vi "CO Serial CAL & Data Recording & DECADEv3.3_test.vi"() -> ()   [LabVIEW 2014]
uses:
  <vilib>/Platform/TimedLoop/XDataNode/timing_clust.ctl
  <vilib>/Platform/TimedLoop/XDataNode/nitl_modes.ctl
  <vilib>/Platform/TimedLoop/XDataNode/wakeup.ctl
  C:/Program Files (x86)/National Instruments/LabVIEW 2014/examples/Data Communication/Network Streams/Simple Network Streams/support/Network Stream Command.ctl
  <vilib>/Utility/error.llb/whitespace.ctl
  <vilib>/Instr/_visa.llb/VISA Configure Serial Port (Instr).vi
  <vilib>/Utility/tcp.llb/UDP Multicast Write-Only Open.vi
  <vilib>/platform/TimedLoop/XDataNode/XDataNode.xnode
  <vilib>/Platform/TimedLoop/XDataNode/XDNodeRunTimeDep.lvlib
panel:
  out "Stop File Write":bool
  out "Default file name":string
  in  "Flight Number 2":string="XXXX"
  out "status":bool
  out "CO Vacuum":bool
  out "CO CAL":bool
  out "error out":errorcluster
  out "CO Vacuum?":i16
  out "Control data":i32[](array[numeric])
  out "Control data out":string
  in  "VISA resource name":refnum<visa-resource-name>="ASRL8::INSTR"
  out "Serial VISA error":errorcluster
  out "SEPTIC TCP Error Out":errorcluster
  out "TCP packet\nSend To SEPTIC":bool
  in  "msec to wait":u32=330 caption="mSec to Wait"
  in  "UDP Time Stamp\nOffset":u32=1
  out "Scan from String Error \nCounter from process loop":i32
  out "TCP Binary Packet":string
  in  "ue9LJ temp":u16
  out "FISH TCP Error Out":errorcluster
  out "TCP packet\nSend To FISH":bool
  out "UDP_Out_Error Out":errorcluster
  out "Data Array":string[](array[string])
  out "UDP_Out Status":bool
  out "Data Process Status":bool
  out "Command In":string[](array[string])
  out "ERR Counter":i32
  out "UDP_Out":string
  out "UDP_Pack_num":u32
  out "Flight Number":string
  in  "aux":string="0"
  in  "acs2653pc_hdd":string="0"
  in  "LabviewVIclient vn":string="0"
  in  "LabviewVIserver vn":string="0"
  in  "PTP Sync":string="0"
  out "OK RAW COUNTER":i32
  out "IN_CAL?":bool
  out "Redundent DATA":string
  out "Data String":string
  out "CO_Data_Buffer":string[](array[string])
  out "RAW DATA":string
  out "loop count":i32
  out "Number of Read error":i32
  out "Command In":string
  # "Pre-flight"
  # "CONC"
  # "SIG"
  # "SENS"
  # "ZERO"
  # "Lamp flow controller"
  # "Lamp temperature"
  # "Monochromater flow controller"
  # "Monochromater temperature"
  # "Monochromater pressure"
  # "Fluorescence cell pressure"
  # "Calibration gas pressure"
  # "Cell temperature"
  # "Calibration Concentration"
  # "ERROR number"
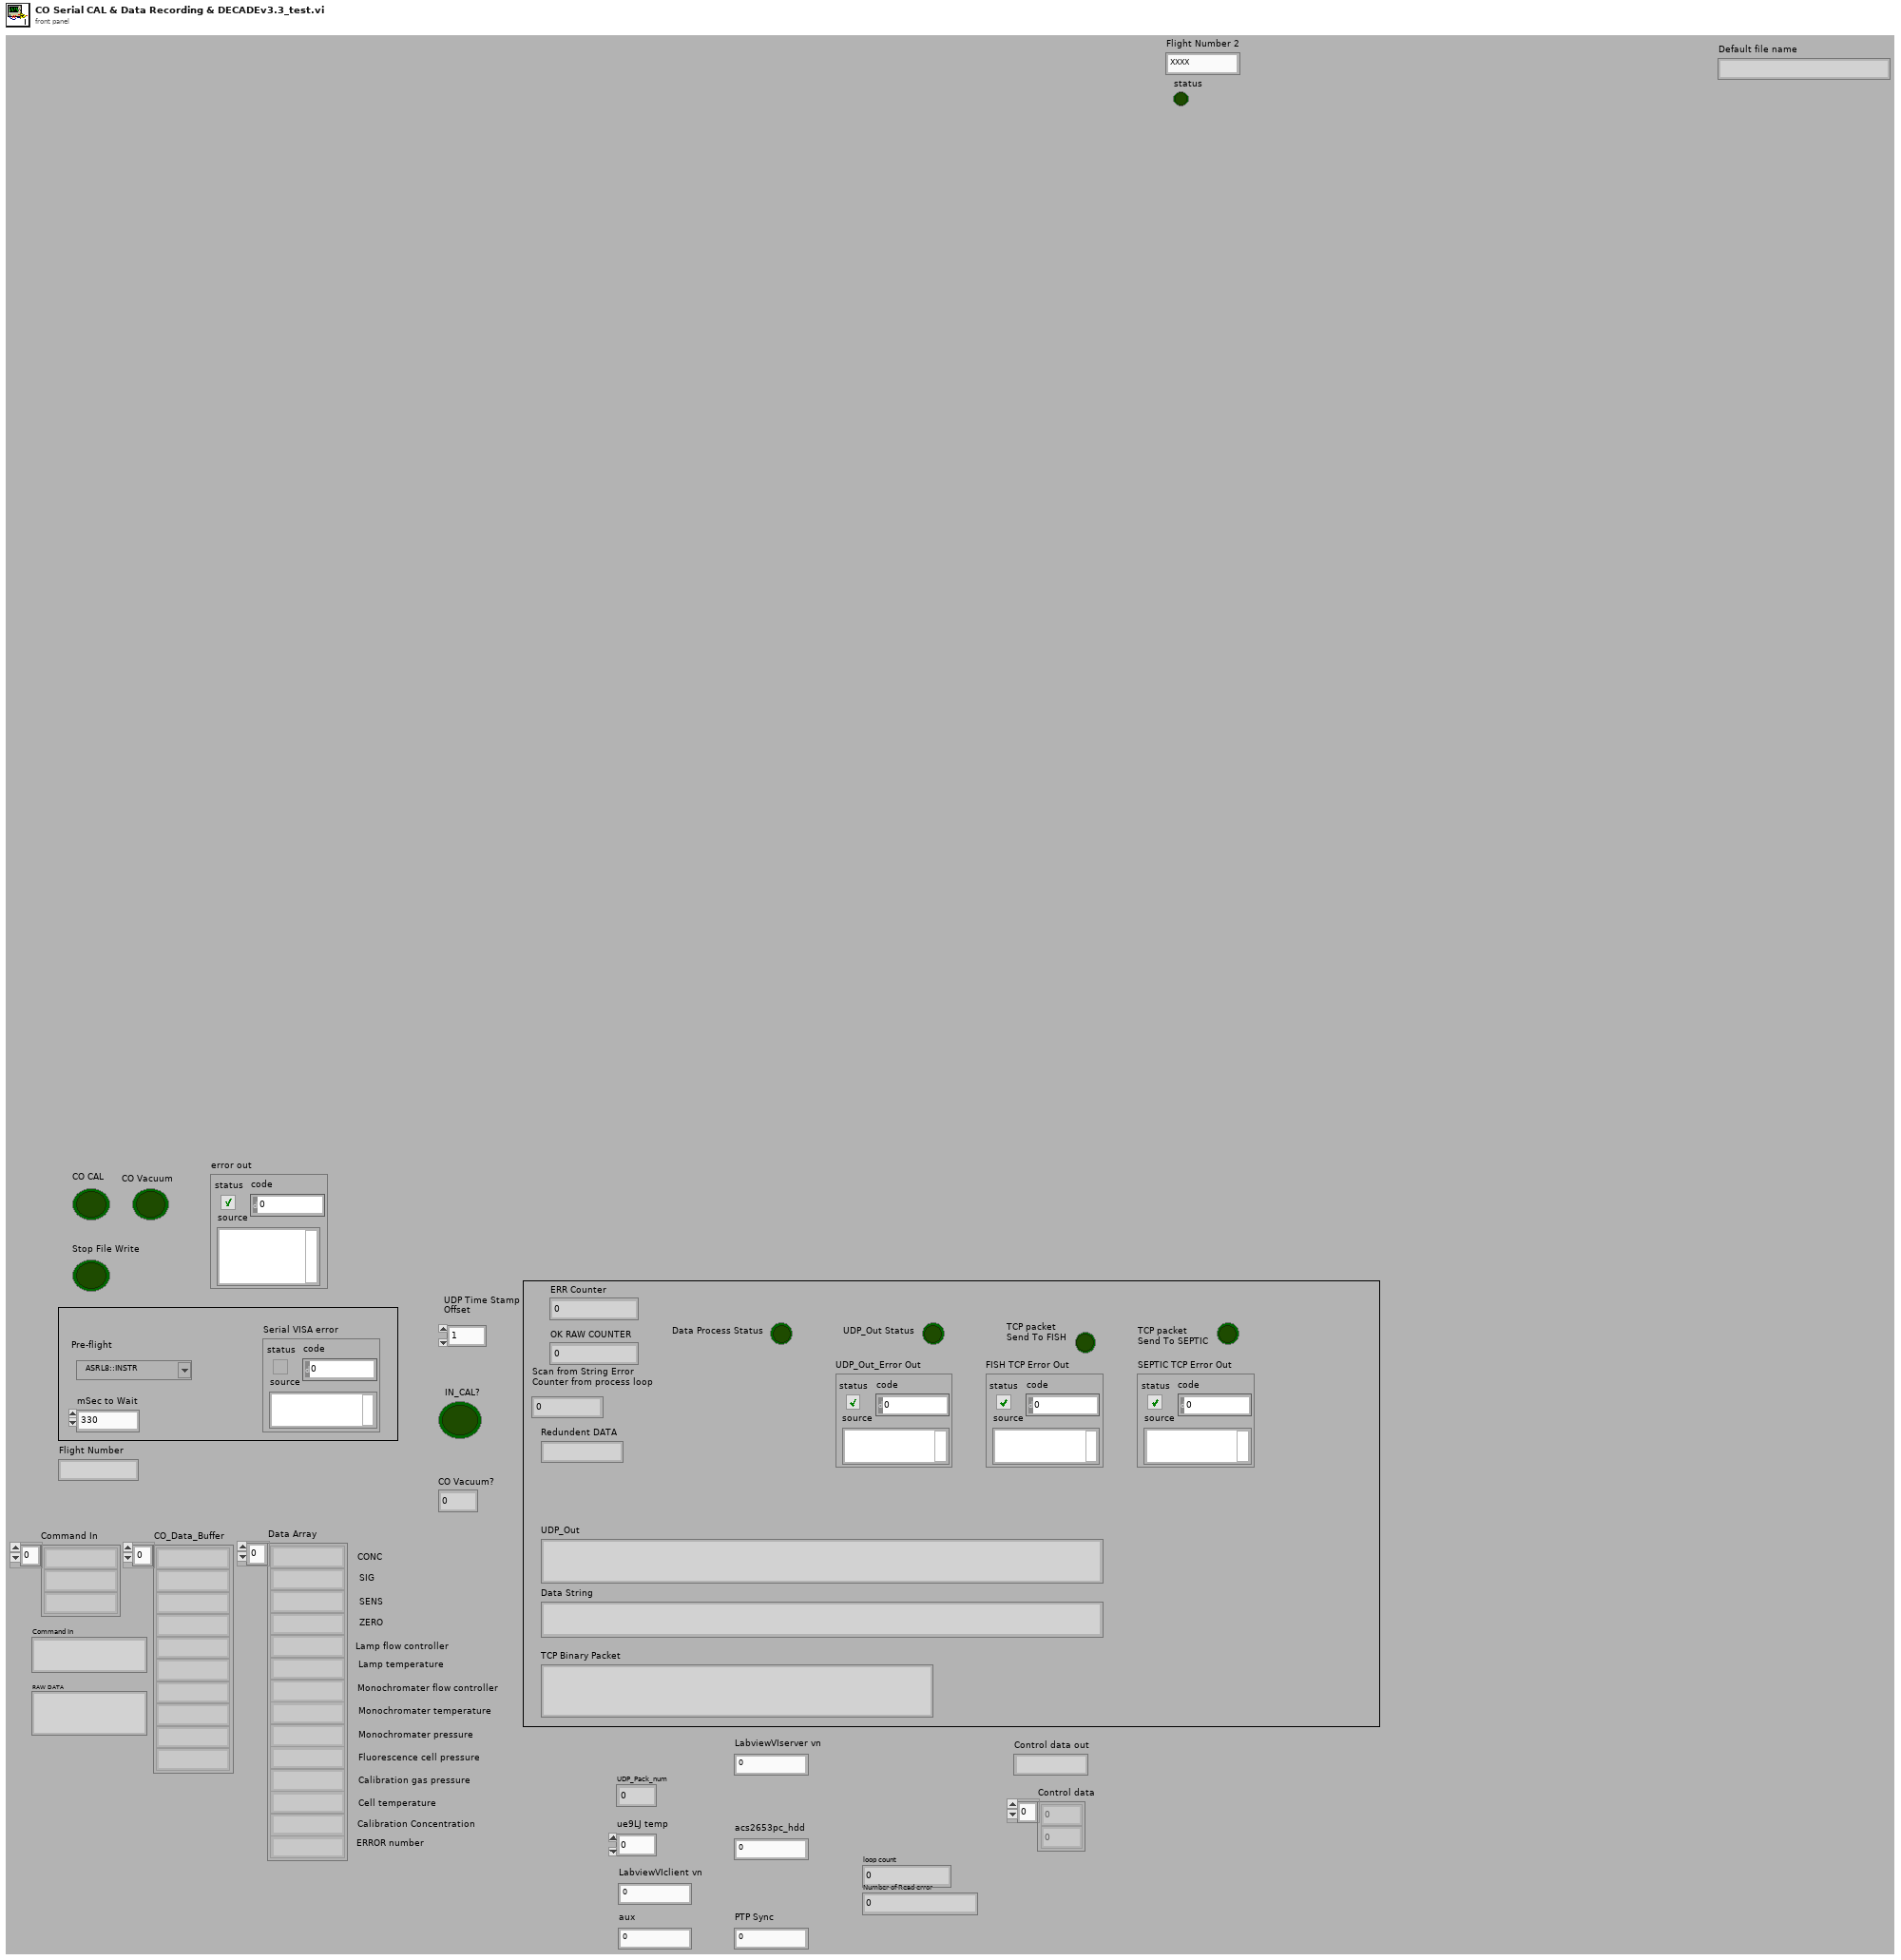
[diagram p1: front panel]
types:
  T1 = typedef "XDNodeRunTimeDep.lvlib/timing_clust.ctl" = cluster{"Expected End [f-1]":u64, "Actual End [f-1]":u64, "Finished Late? [f-1]":bool, "Expected End [i-1]":u64, "Actual End [i-1]":u64, "Finished Late? [i-1]":bool, "Expected Start [i]":u64, "Actual Start [i]":u64, "Expected Start [f]":u64, "Actual Start [f]":u64, "Source Name":string, "Structure Name":string, "Period":i64, "Deadline":i64, "Offset":i64, "Start":i64, "Priority":i32, "Timeout":i32, "Mode":T2, "Wakeup Reason":T3, "Error":errorcluster, "Source Type":string, "Secondary Source Type":string, "Global End Time":u64, "Global Start Time":u64, "Frame Duration":u64, "Iteration Duration":u64, "Assigned CPU":i32, "I/O Scan Engine Mode":u32}
  T2 = typedef "XDNodeRunTimeDep.lvlib/nitl_modes.ctl" = enum32{"No Change", "Process missed periods, maintain original phase", "Discard missed periods, maintain original phase", "Process missed periods, ignore original phase", "Discard missed periods, ignore original phase"}
  T3 = typedef "XDNodeRunTimeDep.lvlib/wakeup.ctl" = enum32{"Normal", "Aborted", "Asynchronous wakeup", "Timing source error", "Timed loop error", "Timeout"}
  T4 = typedef "Network Stream Command.ctl" = cluster{"Message":string, "Message Data":variant}
  T5 = enum16{"open", "replace", "create", "open or create", "replace or create", "replace or create with confirmation"}
  T6 = typedef "whitespace.ctl" = u16
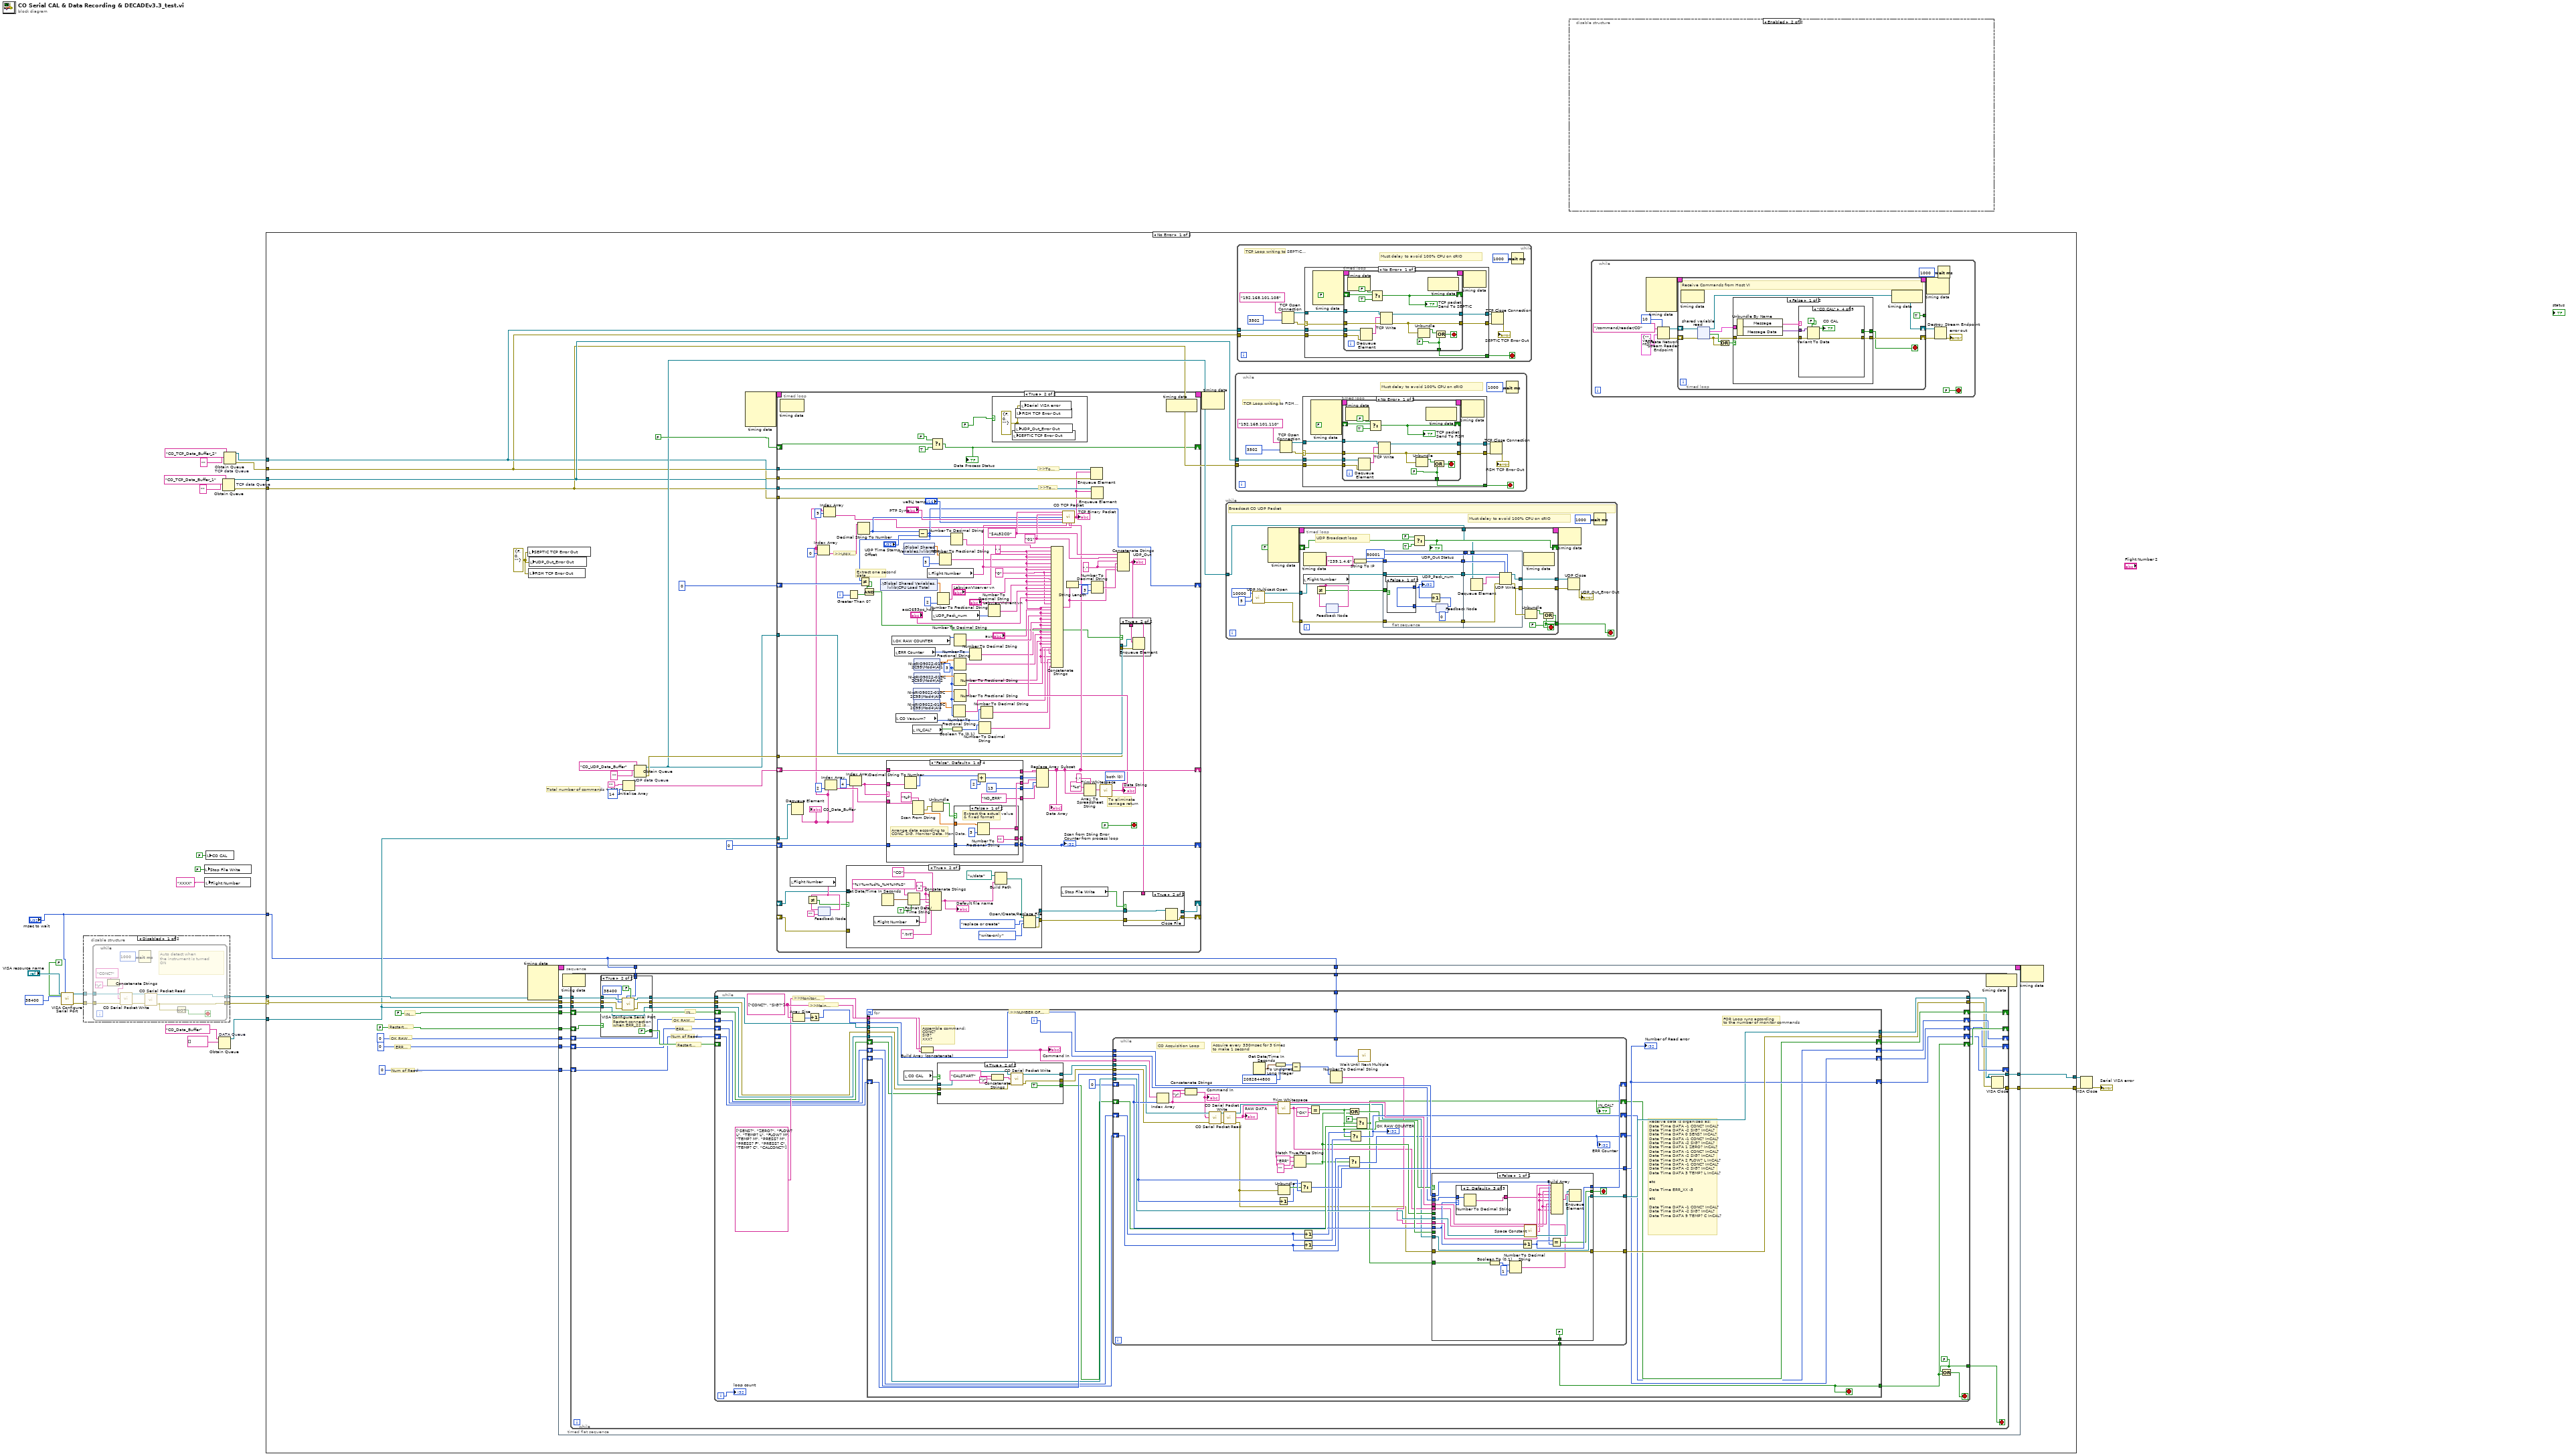
[diagram p0: block diagram]
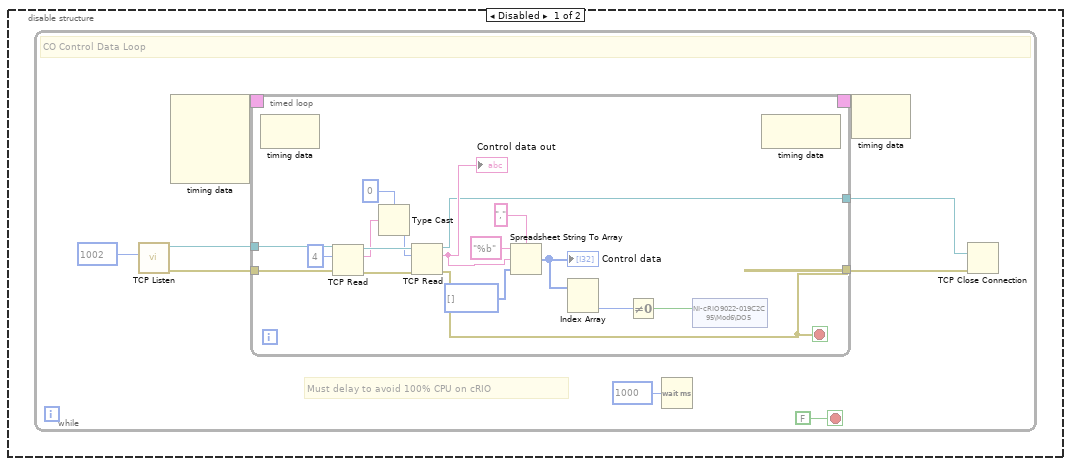
[diagram p3: hidden frame]
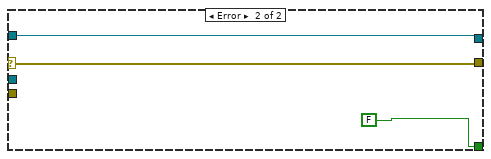
[diagram p4: hidden frame]
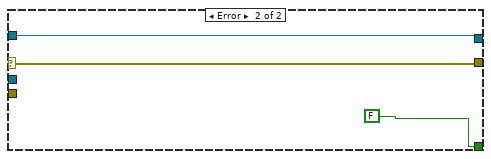
[diagram p5: hidden frame]
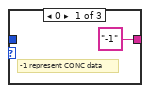
[diagram p7: hidden frame]
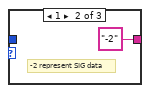
[diagram p8: hidden frame]
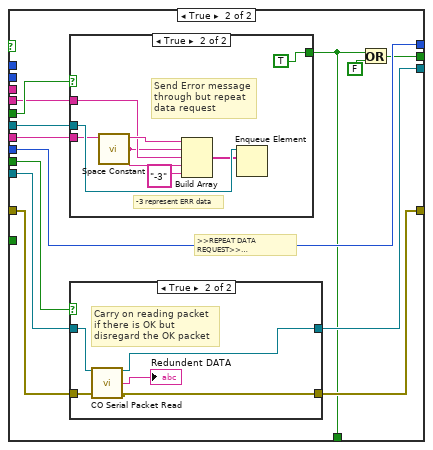
[diagram p9: hidden frame]
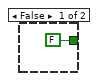
[diagram p11: hidden frame]
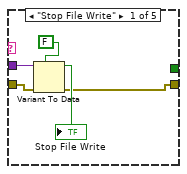
[diagram p13: hidden frame]
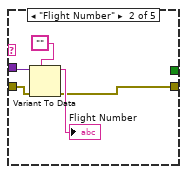
[diagram p14: hidden frame]
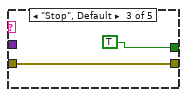
[diagram p15: hidden frame]
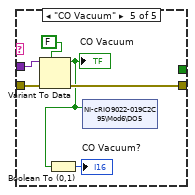
[diagram p16: hidden frame]
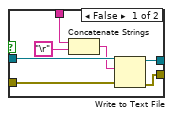
[diagram p19: hidden frame]
diagram:
  n1 = call-poly "VISA Configure Serial Port"("VISA resource name"="VISA resource name", "timeout (10sec)"="msec to wait", "Enable Termination\nChar (T)"=FALSE ("Enable Termination\nChar (T)"), "baud rate (9600)"=u32 38400) -> ("VISA resource name out"=w12:refnum<visa-resource-name>, "error out"=w11:errorcluster)  [unwired: 10 in]
  n2 = disable-structure shown="Disabled" {
    disable-tunnel: w12 -> [w29 _]
    disable-tunnel: w11 -> [w28 _]
    disable-tunnel: [w27 _] -> w10
    disable-tunnel: [w26 _] -> w9
    frame Disabled {
      n3 = while {
        tunnel: w29 -> [w40]
        tunnel: w28 -> [w39]
        tunnel: [w33] -> w27
        tunnel: [w34] -> w26
        stop <- w38 stop-if-true
        # "Auto detect when\nthe instrument is turned \nON"
        n4 = Concatenate Strings("CONC?" ("Data in"), "\r") -> (w30:string)
        n5 = call "CO Serial Packet Write.vi"("VISA resource name In"=w40, "Data in"=w30, "error in (no error)"=w39) -> ("VISA resource name Out"=w36:refnum<visa-resource-name>, "error out"=w35:errorcluster)  [unwired: 11 in]
        n6 = Wait (ms)(milliseconds to wait=u32 1000) -> ()  [unwired: 1 out]
        n7 = call "CO Serial Packet Read.vi"("VISA resource In"=w36, "error in"=w35) -> ("VISA resource Out"=w33:refnum<visa-resource-name>, "error out"=w34:errorcluster)  [unwired: 11 in, 1 out]
        n8 = Not(x=w34) -> (.not. x?=w38:bool)
      }
    }
    frame Enabled {
    }
  }
  n9 = local write "Stop File Write"(FALSE ("Stop File Write")) -> ()
  n10 = local write "Flight Number"("XXXX" ("Flight Number")) -> ()
  n11 = local write "CO CAL"(FALSE ("CO CAL")) -> ()
  n12 = Obtain Queue "DATA Queue"(name (unnamed)="CO_Data_Buffer", element data type=string[] []) -> (queue out=w23:refnum<queue>)  [unwired: 3 in, 2 out]
  n13 = Obtain Queue "TCP data Queue"(name (unnamed)="CO_TCP_Data_Buffer_1", element data type="") -> (queue out=w22:refnum<queue>, error out=w21:errorcluster)  [unwired: 3 in, 1 out]
  n14 = Obtain Queue "TCP data Queue"(name (unnamed)="CO_TCP_Data_Buffer_2", element data type="") -> (queue out=w20:refnum<queue>, error out=w19:errorcluster)  [unwired: 3 in, 1 out]
  n15 = case shown="No Error" w9 {
    selector: w9 -> [w68 w697]
    tunnel: w10 -> [w69 w696]
    tunnel: [w70 w697] -> w15
    tunnel: [w46 w696] -> w14
    tunnel: w23 -> [w67 _]
    tunnel: w22 -> [w56 _]
    tunnel: w21 -> [w55 _]
    tunnel: w20 -> [w54 _]
    tunnel: w19 -> [w53 _]
    tunnel: "msec to wait" -> [w41 _]
    frame No Error {
      w52 = errorcluster {"status"=FALSE, "code"=0, "source"=""} ("UDP_Out_Error Out")
      # "Restart connection?"
      # "IN CAL?"
      # "OK RAW Counter"
      # "ERR Counter"
      # "Num of Read Error"
      # "Total number of commands + ERR"
      n16 = node-c288() -> (w43:T1)  [unwired: 4 in]
      n17 = local write "SEPTIC TCP Error Out"(w52) -> ()
      n18 = local write "FISH TCP Error Out"(w52) -> ()
      n19 = local write "UDP_Out_Error Out"(w52) -> ()
      n20 = timed-sequence {
        timing: w43 -> [_]
        timing-out: [_] -> w42
        tunnel: [w166] -> w70
        tunnel: w69 -> [w165]
        tunnel: w68 -> [w164]
        tunnel: w67 -> [w163]
        tunnel: FALSE -> [w162]
        tunnel: 0 -> [w161]
        tunnel: 0 -> [w160]
        tunnel: 0 -> [w159]
        tunnel: FALSE ("IN_CAL?") -> [w158]
        tunnel: [w157] -> w46
        tunnel: w41 -> [w156]
        tunnel: w41 -> [w155]
        n21 = timed-flat-sequence {
          tunnel: [w178] -> w166
          tunnel: w165 -> [w177]
          tunnel: w164 -> [w176]
          tunnel: w163 -> [w175]
          tunnel: w162 -> [w174]
          tunnel: w161 -> [w173]
          tunnel: w160 -> [w172]
          tunnel: w159 -> [w171]
          tunnel: w158 -> [w170]
          tunnel: [w169] -> w157
          tunnel: w156 -> [w168]
          tunnel: w155 -> [w167]
          n22 = node-c288() -> ()  [unwired: 1 in, 1 out]
          n23 = while {
            tunnel: [w183] -> w178
            tunnel: w177 -> [w200]
            tunnel: w176 -> [w199]
            tunnel: w175 -> [w197]
            shift-right: [w194] -> _
            shift-left: w174 -> [w195]
            shift-right: [w190] -> _
            shift-left: w173 -> [w191]
            shift-right: [w187] -> _
            shift-left: w172 -> [w189]
            shift-right: [w186] -> _
            shift-left: w171 -> [w188]
            shift-right: [w184] -> _
            shift-left: w170 -> [w185]
            tunnel: [w181] -> w169
            tunnel: w168 -> [w180]
            tunnel: w167 -> [w179]
            stop <- w193 stop-if-true
            # "Restart connection?"
            # "Num of Read Error"
            # "ERR Counter"
            # "IN CAL?"
            # "OK RAW Counter"
            n24 = case shown="True" w195 {
              selector: w195 -> [w202 _]
              tunnel: [w205 w211] -> w201
              tunnel: w200 -> [w205 w212]
              tunnel: [w204 w210] -> w198
              tunnel: w199 -> [w204 w209]
              tunnel: [w203 w214] -> w196
              tunnel: w197 -> [w203 w214]
              tunnel: [w202 FALSE] -> w192
              tunnel: w179 -> [_ w206]
              frame False {
              }
              frame True {
                # "Restart connection\nwhen ERR_22 is detected"
                n25 = call-poly "VISA Configure Serial Port"("VISA resource name"=w212, "timeout (10sec)"=w206, "Enable Termination\nChar (T)"=FALSE ("Enable Termination\nChar (T)"), "baud rate (9600)"=u32 38400, "error in (no error)"=w209) -> ("VISA resource name out"=w211:refnum<visa-resource-name>, "error out"=w210:errorcluster)  [unwired: 9 in]
              }
            }
            n26 = while {
              tunnel: [w236] -> w182
              tunnel: w201 -> [w235]
              tunnel: w198 -> [w234]
              tunnel: [w233] -> w181
              tunnel: w196 -> [w232]
              shift-right: [w223] -> w190
              shift-left: w191 -> [w227]
              shift-right: [w222] -> w187
              shift-left: w189 -> [w226]
              shift-right: [w221] -> w184
              shift-left: w185 -> [w225]
              shift-right: [w220] -> w186
              shift-left: w188 -> [w224]
              tunnel: [w216] -> w193
              shift-right: [w217] -> w194
              shift-left: w192 -> [_]
              tunnel: w180 -> [w215]
              i -> [w219]
              stop <- w218 stop-if-true
              w216 = FALSE
              w231 = string[] ["CONC?", "SIG?"]
              # ">>Main commands>>"
              # ">>Monitor Command>>"
              n27 = Array Size(array=w231) -> (size(s)=w228:i32)
              n28 = Increment(x=w228) -> (x+1=w230:i32)
              n29 = for {
                tunnel: w235 -> [w256]
                tunnel: w234 -> [w255]
                tunnel: [w261] -> w236
                shift-right: [w259] -> w220
                shift-left: w224 -> [w260]
                tunnel: [w258] -> w233
                tunnel: w232 -> [w257]
                tunnel: w230 -> [w251]
                shift-right: [w249] -> w221
                shift-left: w225 -> [w250]
                shift-right: [w247] -> w222
                shift-left: w226 -> [w248]
                shift-right: [w245] -> w223
                shift-left: w227 -> [w246]
                tunnel: string[] ["SENS?", "ZERO?", "FLOW? L", "TEMP? L", "FLOW? M", "TEMP? M", "PRESS? M", "PRESS? F", "PRESS? C", "TEMP? C", "CALCONC?"] -> [w242] mode=indexing
                tunnel: w231 -> [w243]
                tunnel: [w240] -> w217
                tunnel: w215 -> [w238]
                i -> [w241]
                stop <- w240 stop-if-true
                # "Receive data is organised as:\nDate Time DATA -1 CONC? InCAL?\nDate Time DATA -2 SIG? InCAL?\nDate Time DATA 0 SENS? InCAL?\nDate Time DATA -1 CONC? InCAL?\nDate Time DATA -2 SIG? InCAL?\nDate Time DATA 1 ZERO? InCAL?\nDate Time DATA -1 CONC? InCAL?\nDate Time DATA -2 SIG? InCAL?\nDate Time DATA 2 FLOW? L InCAL?\nDate Time DATA -1 CONC? InCAL?\nDate Time DATA -2 SIG? InCAL?\nDate Time DATA 3 TEMP? L InCAL?\n\netc\n\nDate Time ERR_XX -3\n\netc\n\nDate Time DATA -1 CONC? InCAL?\nDate Time DATA -2 SIG? InCAL?\nDate Time DATA 9 TEMP? C InCAL?"
                # "FOR Loop runs according\nto the number of monitor commands"
                # "Assemble command:\nCONC?\nSIG?\nXXX?"
                # ">>NUMBER OF COMMANDS>>"
                n30 = local read "CO CAL"() -> (w237:bool)
                n31 = Build Array (concatenate)(w243, w242) -> (w244:string[])
                "Command In" <- w244
                n32 = case shown="True" w237 {
                  tunnel: w256 -> [w361 w363]
                  tunnel: w255 -> [w360 w366]
                  tunnel: [w361 w364] -> w254
                  tunnel: [w360 w365] -> w253
                  tunnel: [w359 TRUE ("IN_CAL?")] -> w252
                  tunnel: w250 -> [w359 _]
                  frame False {
                  }
                  frame True {
                    n33 = Concatenate Strings("CALSTART" ("string"), "\r") -> (w362:string)
                    n34 = call "CO Serial Packet Write.vi"("VISA resource name In"=w363, "Data in"=w362, "error in (no error)"=w366) -> ("VISA resource name Out"=w364:refnum<visa-resource-name>, "error out"=w365:errorcluster)  [unwired: 11 in]
                  }
                }
                n35 = while {
                  tunnel: w253 -> [w268]
                  tunnel: [w295] -> w261
                  tunnel: w260 -> [w307]
                  tunnel: [w306] -> w259
                  tunnel: w244 -> [w299]
                  tunnel: [w296] -> w258
                  tunnel: w257 -> [w294]
                  tunnel: w254 -> [w270]
                  shift-right: [w271] -> w249
                  shift-left: w252 -> [w301]
                  shift-right: [w298] -> _
                  shift-left: 0 -> [w300]
                  tunnel: w251 -> [w291]
                  shift-right: [w288] -> w247
                  shift-left: w248 -> [w289]
                  shift-right: [w282] -> w245
                  shift-left: w246 -> [w284]
                  tunnel: w241 -> [w281]
                  tunnel: [w276] -> w240
                  tunnel: w238 -> [w262]
                  stop <- w297 stop-if-true
                  # "Acquire every 330msec for 3 times\nto make 1 second"
                  # "CO Acquisition Loop"
                  n36 = Index Array(array=w299, index=w300) -> (element=w293:string)
                  n37 = Concatenate Strings(w293, "\r") -> (w269:string)
                  "Command In" <- w269
                  n38 = call "CO Serial Packet Write.vi"("VISA resource name In"=w270, "Data in"=w269, "error in (no error)"=w268) -> ("VISA resource name Out"=w266:refnum<visa-resource-name>, "error out"=w267:errorcluster)  [unwired: 11 in]
                  n39 = call "CO Serial Packet Read.vi"("VISA resource In"=w266, "error in"=w267) -> ("VISA resource Out"=w265:refnum<visa-resource-name>, "Data Out"=w263:string, "error out"=w264:errorcluster)  [unwired: 11 in]
                  "RAW DATA" <- w263
                  n40 = Get Date/Time In Seconds() -> (seconds since 1Jan1904=w277:timestamp)
                  n41 = To Unsigned Long Integer(number=w277) -> (unsigned 32bit integer=w280:u32)
                  n42 = Increment(x=w307) -> (x+1=w303:i32)
                  n43 = call <vilib>:"Trim Whitespace.vi"("string"=w263) -> ("trimmed string"=w275:string)  [unwired: 1 in]
                  n44 = Unbundle(w264) -> ("status"=w304:bool)  [unwired: 2 out]
                  n45 = Subtract(x=w280, y=u32 2082844800) -> (x-y=w272:u32)
                  n46 = Match True/False String(2:"" ("false string"), 3:"ERR" ("true string"), 4:w263) -> (0:w283:bool)  [unwired: 1 out]
                  n47 = Select(t=w303, s=w304, f=w307) -> (s? t:f=w306:i32)
                  n48 = Increment(x=w289) -> (x+1=w290:i32)
                  n49 = Increment(x=w284) -> (x+1=w285:i32)
                  n50 = Equal?(x=w275, y="OK" ("string")) -> (x = y?=w286:bool)
                  n51 = Number To Decimal String(number=w272) -> (decimal integer string=w278:string)  [unwired: 1 in]
                  n52 = Select(t=w285, s=w283, f=w284) -> (s? t:f=w282:i32)
                  "ERR Counter" <- w282
                  n53 = Select(t=w290, s=w286, f=w289) -> (s? t:f=w288:i32)
                  "OK RAW COUNTER" <- w288
                  n54 = Compound Arithmetic op=OR(w286, w283) -> (w287:bool)
                  n55 = Select(t=FALSE, s=w286, f=w301) -> (s? t:f=w271:bool)
                  "IN_CAL?" <- w271
                  n56 = call "Wait Until Next Multiple"("Count(mSec)"=w262) -> ()  [unwired: 1 out]
                  n57 = case shown="False" w287 {
                    tunnel: w300 -> [w315 w343]
                    tunnel: [w326 w343] -> w298
                    tunnel: [w320 w333] -> w297
                    tunnel: w265 -> [w325 w342]
                    tunnel: w264 -> [w324 w341]
                    tunnel: [w325 w340] -> w296
                    tunnel: [w324 w339] -> w295
                    tunnel: w294 -> [w322 w337]
                    tunnel: w275 -> [w313 w335]
                    tunnel: w293 -> [w316 _]
                    tunnel: w278 -> [w321 w336]
                    tunnel: w283 -> [_ w338]
                    tunnel: w291 -> [w319 _]
                    tunnel: w286 -> [_ w334]
                    tunnel: w281 -> [w318 _]
                    tunnel: [FALSE w331] -> w276
                    tunnel: w271 -> [w312 _]
                    frame False {
                      n58 = case shown="2, Default" w315 {
                        tunnel: w318 -> [_ _ w330]
                        tunnel: ["-1" "-2" w329] -> w317
                        frame 0 {
                          # "-1 represent CONC data"
                        }
                        frame 1 {
                          # "-2 represent SIG data"
                        }
                        frame 2, Default {
                          n59 = Number To Decimal String(number=w330) -> (decimal integer string=w329:string)  [unwired: 1 in]
                        }
                      }
                      n60 = Boolean To (0,1)(Boolean=w312) -> (0, 1=w311:i16)
                      n61 = Number To Decimal String(number=w311, width (-)=i16 1) -> (decimal integer string=w308:string)
                      n62 = Increment(x=w315) -> (x+1=w326:i32)
                      n63 = call <vilib>:"Space Constant.vi"() -> ("String"=w309:string)
                      n64 = Equal?(x=w326, y=w319) -> (x = y?=w320:bool)
                      n65 = Build Array(w321, w309, w313, w309, w317, w309, w316, w313, w309, w308) -> (w323:string[])
                      n66 = Enqueue Element(queue=w322, element=w323) -> ()  [unwired: 2 in, 3 out]
                    }
                    frame True {
                      # ">>REPEAT DATA REQUEST>>\nif OK or ERR"
                      n67 = case shown="True" w338 {
                        tunnel: w337 -> [_ w358]
                        tunnel: w336 -> [_ w356]
                        tunnel: w335 -> [_ w355]
                        tunnel: [FALSE TRUE] -> w331
                        frame False {
                        }
                        frame True {
                          # "-3 represent ERR data"
                          # "Send Error message\nthrough but repeat\ndata request"
                          n68 = call <vilib>:"Space Constant.vi"() -> ("String"=w354:string)
                          n69 = Build Array(w356, w354, w355, w354, "-3" ("element")) -> (w357:string[])
                          n70 = Enqueue Element(queue=w358, element=w357) -> ()  [unwired: 2 in, 3 out]
                        }
                      }
                      n71 = case shown="True" w334 {
                        tunnel: w342 -> [w344 w349]
                        tunnel: w341 -> [w345 w350]
                        tunnel: [w344 w348] -> w340
                        tunnel: [w345 w346] -> w339
                        frame False {
                        }
                        frame True {
                          # "Carry on reading packet\nif there is OK but\ndisregard the OK packet"
                          n72 = call "CO Serial Packet Read.vi"("VISA resource In"=w349, "error in"=w350) -> ("VISA resource Out"=w348:refnum<visa-resource-name>, "Data Out"=→"Redundent DATA":string, "error out"=w346:errorcluster)  [unwired: 11 in]
                        }
                      }
                      n73 = Or(x=w331, y=FALSE) -> (x .or. y?=w333:bool)
                    }
                  }
                }
                "Number of Read error" <- w259
              }
              n74 = Or(x=w216, y=w217) -> (x .or. y?=w218:bool)
              "loop count" <- w219
            }
            n75 = VISA Close(VISA resource name=w181, error in (no error)=w182) -> (error out=w183:errorcluster)
          }
          n76 = node-c288() -> ()  [unwired: 1 in, 1 out]
        }
      }
      n77 = Initialize Array("", 14) -> (w64:string[])
      n78 = Obtain Queue "UDP data Queue"(name (unnamed)="CO_UDP_Data_Buffer", element data type="") -> (queue out=w59:refnum<queue>, error out=w60:errorcluster)  [unwired: 3 in, 1 out]
      n79 = node-c288() -> (w45:T1)  [unwired: 4 in]
      n80 = timed-loop {
        tunnel: w67 -> [w530]
        shift-right: [w495] -> _
        shift-left: w64 -> [w513]
        shift-right: [w500] -> _
        shift-left: FALSE -> [w503]
        tunnel: w56 -> [w494]
        tunnel: w55 -> [w493]
        tunnel: w59 -> [w491]
        tunnel: w60 -> [w490]
        shift-right: [w488] -> _
        shift-left: 0 -> [w489]
        shift-right: [w474] -> _
        shift-left: 0 -> [w482]
        tunnel: w54 -> [w480]
        tunnel: w53 -> [w479]
        timing: w45 -> [_]
        timing-out: [_] -> w44
        shift-right: [w450] -> _
        shift-left: _ -> [w443]
        shift-right: [w441] -> _
        shift-left: _ -> [w442]
        i -> [w485]
        stop <- FALSE stop-if-true
        w431 = "0" ("string")
        w465 = i16 3 ("precision (6)")
        w505 = T6 0 items=["both", "start of string", "end of string"] ("location (both)")
        w438 = ","
        w498 = "01"
        w516 = ","
        w499 = "$AL52CO"
        # ">>To SEPTIC>>"
        # ">>To FISH>>"
        # "Extract one second data\nfor UDP sending"
        # ">>UNIX TIME>>"
        # "To eliminate\ncarriage return"
        n81 = node-c288() -> ()  [unwired: 1 in, 1 out]
        n82 = local read "Flight Number"() -> (w448:string)
        n83 = Dequeue Element(queue=w530) -> (element=w470:string[])  [unwired: 2 in, 3 out]
        "CO_Data_Buffer" <- w470
        n84 = Index Array(array=w470, index=0) -> (element=w483:string)
        n85 = feedback #1("" ("Flight Number")) -> (w447:string)
        n86 = Not Equal?(x=w448, y=w447) -> (x != y?=w446:bool)
        n87 = feedback-in #1(w448) -> ()
        n88 = Index Array(array=w470, index=9) -> (element=w469:string)
        n89 = Index Array(array=w470, index=2) -> (element=w511:string)
        n90 = case shown="True" w446 {
          tunnel: [w532 w534] -> w445
          tunnel: [w531 w533] -> w444
          tunnel: w443 -> [w532 _]
          tunnel: w442 -> [w531 _]
          frame False {
          }
          frame True {
            w541 = "_" ("string")
            n91 = local read "Flight Number"() -> (w547:string)
            n92 = Get Date/Time In Seconds() -> (seconds since 1Jan1904=w542:timestamp)
            n93 = Format Date/Time String(time format string (%c)="%Y%m%d%_%H%M%S", seconds (now)=w542, UTC format=TRUE) -> (date/time string=w545:string)
            n94 = Concatenate Strings("CO" ("string"), w541, w545, w541, w547, ".txt" ("string")) -> (w539:string)
            "Default file name" <- w539
            n95 = Build Path(base path=path "u:/data", name or relative path=w539) -> (appended path=w535:path)
            n96 = Open/Create/Replace File(file path (use dialog)=w535, operation (0:open)=T5."replace or create", access (0:read/write)=enum16{"read/write", "read-only", "write-only"}."write-only") -> (refnum out=w534:refnum<file>, error out=w533:errorcluster)  [unwired: 3 in, 1 out]
          }
        }
        n97 = Greater Than 0?(x=w485) -> (x > 0?=w484:bool)
        n98 = Index Array(array=w470, index=4) -> (element=w512:string)
        n99 = Decimal String To Number(string=w483) -> (number=w477:i32)  [unwired: 2 in, 1 out]
        n100 = shared-variable ".\\Global Shared Variables.lvlib\\CPU Load Total"() -> (w437:dbl)  [unwired: 1 in, 1 out]
        n101 = case shown="\"False\", Default" w512 {
          tunnel: w512 -> [w578 _ _ _]
          tunnel: w513 -> [w579 w601 w623 w637]
          tunnel: w511 -> [w570 w595 w617 w633]
          tunnel: [w579 w601 w623 w637] -> w510
          tunnel: [w576 0 ("index") 1 ("index") w634] -> w509
          tunnel: [w569 w591 w613 w633] -> w508
          tunnel: [w568 w592 w614 ""] -> _
          tunnel: w489 -> [w567 w594 w616 w635]
          tunnel: [w566 w593 w615 w635] -> w488
          tunnel: [13 ("index") 13 ("index") 13 ("index") w634] -> w473
          tunnel: ["NO_ERR" "NO_ERR" "NO_ERR" w633] -> w472
          frame "False", Default {
            # "Arrange data according to\nCONC, SIG, Monitor Data, Mon Data,"
            n102 = Decimal String To Number(string=w578) -> (number=w575:i32)  [unwired: 2 in, 1 out]
            n103 = Scan From String(format string="%f", input string=w570) -> (error out=w572:errorcluster, output 1=w573:dbl)  [unwired: 3 in, 2 out]
            n104 = Unbundle(w572) -> ("status"=w571:bool)  [unwired: 2 out]
            n105 = case shown="False" w571 {
              tunnel: [w584 ""] -> w569
              tunnel: w573 -> [w583 _]
              tunnel: w567 -> [w582 w587]
              tunnel: [w582 w586] -> w566
              tunnel: ["" "Scan from string error"] -> w568
              frame False {
                # "Extract the actual value\n& fixed format"
                n106 = Number To Fractional String(number=w583, precision (6)=i16 3) -> (F-format string=w584:string)  [unwired: 2 in]
              }
              frame True {
                # "If scan from string error,\nreplace data with empty\nstring"
                n107 = Increment(x=w587) -> (x+1=w586:i32)
              }
            }
            n108 = Add(x=w575, y=2) -> (x+y=w576:i32)
          }
          frame "-1" {
            # "Arrange data according to\nCONC, SIG, Monitor Data, Mon Data,"
            # "-1 represent CONC data"
            n109 = Scan From String(format string="%f", input string=w595) -> (error out=w597:errorcluster, output 1=w598:dbl)  [unwired: 3 in, 2 out]
            n110 = Unbundle(w597) -> ("status"=w596:bool)  [unwired: 2 out]
            n111 = case shown="False" w596 {
              tunnel: [w606 ""] -> w591
              tunnel: w598 -> [w605 _]
              tunnel: w594 -> [w604 w609]
              tunnel: [w604 w608] -> w593
              tunnel: ["" "Scan from string error"] -> w592
              frame False {
                # "Extract the actual value\n& fixed format"
                n112 = Number To Fractional String(number=w605, precision (6)=i16 5) -> (F-format string=w606:string)  [unwired: 2 in]
              }
              frame True {
                # "If scan from string error,\nreplace data with empty\nstring"
                n113 = Increment(x=w609) -> (x+1=w608:i32)
              }
            }
          }
          frame "-2" {
            # "Arrange data according to\nCONC, SIG, Monitor Data, Mon Data,"
            # "-2 represent SIG data"
            n114 = Scan From String(format string="%f", input string=w617) -> (error out=w619:errorcluster, output 1=w620:dbl)  [unwired: 3 in, 2 out]
            n115 = Unbundle(w619) -> ("status"=w618:bool)  [unwired: 2 out]
            n116 = case shown="False" w618 {
              tunnel: [w628 ""] -> w613
              tunnel: w620 -> [w627 _]
              tunnel: w616 -> [w626 w631]
              tunnel: [w626 w630] -> w615
              tunnel: ["" "Scan from string error"] -> w614
              frame False {
                # "Extract the actual value\n& fixed format"
                n117 = Number To Fractional String(number=w627, precision (6)=i16 3) -> (F-format string=w628:string)  [unwired: 2 in]
              }
              frame True {
                # "If scan from string error,\nreplace data with empty\nstring"
                n118 = Increment(x=w631) -> (x+1=w630:i32)
              }
            }
          }
          frame "-3" {
            w634 = 13 ("index")
            # "-3 represent ERR data"
          }
        }
        "Scan from String Error \nCounter from process loop" <- w488
        n119 = local read "OK RAW COUNTER"() -> (w514:i32)
        n120 = local read "ERR Counter"() -> (w453:i32)
        n121 = local read "CO Vacuum?"() -> (w456:i16)
        n122 = shared-variable ".\\Global Shared Variables.lvlib\\MFM"() -> (w436:dbl)  [unwired: 1 in, 1 out]
        n123 = local read "IN_CAL?"() -> (w464:bool)
        n124 = shared-variable "NI-cRIO9022-019C2C95\\Mod4\\AI3"() -> (w462:dbl)  [unwired: 1 in, 1 out]
        n125 = shared-variable "NI-cRIO9022-019C2C95\\Mod4\\AI4"() -> (w461:dbl)  [unwired: 1 in, 1 out]
        n126 = shared-variable "NI-cRIO9022-019C2C95\\Mod4\\AI1"() -> (w467:dbl)  [unwired: 1 in, 1 out]
        n127 = shared-variable "NI-cRIO9022-019C2C95\\Mod4\\AI2"() -> (w466:dbl)  [unwired: 1 in, 1 out]
        n128 = Subtract(x=w477, y="UDP Time Stamp\nOffset") -> (x-y=w474:u32)
        n129 = Not Equal?(x=w474, y=w482) -> (x != y?=w486:bool)
        n130 = Compound Arithmetic op=AND(w486, w484) -> (w481:bool)
        n131 = local read "Flight Number"() -> (w440:string)
        n132 = Select(t=FALSE, s=w503, f=TRUE) -> (s? t:f=w500:bool)
        "Data Process Status" <- w500
        n133 = local read "UDP_Pack_num"() -> (w524:u32)
        n134 = Number To Fractional String(number=w437, precision (6)=i16 2 ("width (-)")) -> (F-format string=w433:string)  [unwired: 2 in]
        n135 = Number To Fractional String(number=w436, precision (6)=i16 3 ("width (-)")) -> (F-format string=w432:string)  [unwired: 2 in]
        n136 = Number To Decimal String(number=w474) -> (decimal integer string=w475:string)  [unwired: 1 in]
        n137 = Boolean To (0,1)(Boolean=w464) -> (0, 1=w463:i16)
        n138 = Number To Fractional String(number=w461, precision (6)=w465) -> (F-format string=w457:string)  [unwired: 2 in]
        n139 = Number To Fractional String(number=w467, precision (6)=w465) -> (F-format string=w460:string)  [unwired: 2 in]
        n140 = Number To Fractional String(number=w466, precision (6)=w465) -> (F-format string=w459:string)  [unwired: 2 in]
        n141 = Number To Fractional String(number=w462, precision (6)=w465) -> (F-format string=w458:string)  [unwired: 2 in]
        n142 = Number To Decimal String(number=w514) -> (decimal integer string=w520:string)  [unwired: 1 in]
        n143 = Number To Decimal String(number=w453) -> (decimal integer string=w452:string)  [unwired: 1 in]
        n144 = Number To Decimal String(number=w463) -> (decimal integer string=w454:string)  [unwired: 1 in]
        n145 = Number To Decimal String(number=w456) -> (decimal integer string=w455:string)  [unwired: 1 in]
        n146 = Number To Decimal String(number=w524) -> (decimal integer string=w523:string)  [unwired: 1 in]
        n147 = case shown="True" FALSE {
          frame False {
          }
          frame True {
            w560 = errorcluster {"status"=FALSE, "code"=0, "source"=""} ("UDP_Out_Error Out")
            n148 = local write "SEPTIC TCP Error Out"(w560) -> ()
            n149 = local write "UDP_Out_Error Out"(w560) -> ()
            n150 = local write "FISH TCP Error Out"(w560) -> ()
            n151 = local write "Serial VISA error"(w560) -> ()
          }
        }
        n152 = Replace Array Subset(array=w510, new element #1=w508, index #1=w509, new element #2=w472, index #2=w473) -> (w495:string[])
        "Data Array" <- w495
        n153 = local read "Stop File Write"() -> (w449:bool)
        n154 = call "CO TCP Packet.vi"("ID"=w499, "Version"=w498, "utc_time"=w477, "PTP Sync"="PTP Sync", "ue9LJ temp"="ue9LJ temp", "Flight Number"=w440, "Data Array"=w495, "In_CAL?"=w469) -> ("TCP Binary Packet"=w478:string)  [unwired: 7 in]
        "TCP Binary Packet" <- w478
        n155 = Array To Spreadsheet String(delimiter (Tab)=",", array=w495, 3:"%s" ("format string")) -> (spreadsheet string=w504:string)
        n156 = Enqueue Element(queue=w480, element=w478, error in (no error)=w479) -> ()  [unwired: 1 in, 3 out]
        n157 = Enqueue Element(queue=w494, element=w478, error in (no error)=w493) -> ()  [unwired: 1 in, 3 out]
        n158 = call <vilib>:"Trim Whitespace.vi"("string"=w504, "location (both)"=w505) -> ("trimmed string"=w492:string)
        "Data String" <- w492
        n159 = Concatenate Strings(w475, w438, w433, w438, w432, w438, w440, w438, w431, w438, "LabviewVIserver vn", w438, "LabviewVIclient vn", w438, w523, w438, "acs2653pc_hdd", w438, w431, w438, "aux", w438, w492, w438, w520, w438, w452, w438, w460, w438, w459, w438, w458, w438, w457, w438, w455, w438, w454) -> (w515:string)
        n160 = String Length(string=w515) -> (length=w519:i32)
        n161 = Number To Decimal String(number=w519, width (-)=i16 3) -> (decimal integer string=w517:string)
        n162 = Concatenate Strings(w499, w498, w516, w517, w516, w515) -> (w451:string)
        "UDP_Out" <- w451
        n163 = case shown="True" w481 {
          tunnel: w451 -> [_ w563]
          tunnel: w491 -> [_ w562]
          tunnel: w490 -> [_ w561]
          frame False {
          }
          frame True {
            n164 = Enqueue Element(queue=w562, element=w563, error in (no error)=w561) -> ()  [unwired: 1 in, 3 out]
          }
        }
        n165 = case shown="True" w449 {
          tunnel: w451 -> [w552 _]
          tunnel: w445 -> [w554 w557]
          tunnel: w444 -> [w553 w556]
          tunnel: [w549 _] -> w450
          tunnel: [w548 w555] -> w441
          frame False {
            n166 = Concatenate Strings(w552, "\r") -> (w550:string)
            n167 = Write to Text File(file (use dialog)=w554, text=w550, error in=w553) -> (refnum out=w549:refnum<file>, error out=w548:errorcluster)  [unwired: 2 out]
          }
          frame True {
            n168 = Close File(refnum=w557, error in=w556) -> (error out=w555:errorcluster)  [unwired: 1 out]
          }
        }
        n169 = node-c288() -> ()  [unwired: 1 in, 1 out]
      }
      n170 = node-c288(w44) -> ()  [unwired: 1 out]
      n171 = while {
        tunnel: w59 -> [w641]
        stop <- w642 stop-if-true
        # "Must delay to avoid 100% CPU on cRIO"
        # "Broadcast CO UDP Packet"
        n172 = call-poly <vilib>:"UDP Multicast Open.vi"("time-to-live (1)"=u16 5, "port"=u16 10000) -> ("error out"=w649:errorcluster, "connection ID"=w650:refnum<k16>)  [unwired: 8 in]
        n173 = node-c288() -> (w652:T1)  [unwired: 4 in]
        n174 = timed-loop {
          tunnel: w650 -> [w672]
          tunnel: w649 -> [w671]
          timing: w652 -> [_]
          timing-out: [_] -> w651
          shift-right: [w659] -> _
          shift-left: FALSE -> [w662]
          tunnel: [w658] -> w644
          tunnel: [w656] -> w643
          tunnel: [w654] -> w642
          tunnel: w641 -> [w653]
          stop <- w655 stop-if-true
          w654 = FALSE
          # "UDP Broadcast loop"
          n175 = node-c288() -> ()  [unwired: 1 in, 1 out]
          n176 = local read "Flight Number"() -> (w665:string)
          n177 = feedback-in #2(w665) -> ()
          n178 = feedback #2() -> (w664:string)  [unwired: 1 in]
          n179 = Not Equal?(x=w665, y=w664) -> (x != y?=w663:bool)
          n180 = String To IP(1:"239.1.4.6" ("name")) -> (0:w669:u32)
          n181 = flat-sequence {
            tunnel: w669 -> [w679]
            tunnel: w671 -> [w680]
            tunnel: w672 -> [w681]
            tunnel: [w681] -> w668
            tunnel: [w680] -> w667
            tunnel: [w679] -> w666
            tunnel: w663 -> [w678]
            tunnel: u16 50001 ("port or service name") -> [w691]
            tunnel: w668 -> [w690]
            tunnel: w667 -> [w689]
            tunnel: w666 -> [w688]
            tunnel: [w687] -> w658
            tunnel: [w686] -> w656
            tunnel: w653 -> [w684]
            frame #0 {
              n182 = feedback #3(u32 0) -> (w675:u32)
              n183 = case shown="False" w678 {
                tunnel: w675 -> [w682 _]
                tunnel: [w682 u32 0] -> w674
                frame False {
                }
                frame True {
                }
              }
              "UDP_Pack_num" <- w674
              n184 = Increment(x=w674) -> (x+1=w676:u32)
              n185 = feedback-in #3(w676) -> ()
            }
            frame #1 {
              n186 = Dequeue Element(queue=w684) -> (element=w685:string)  [unwired: 2 in, 3 out]
              n187 = UDP Write(address=w688, port or service name=w691, connection ID=w690, data in=w685, 8:w689) -> (error out=w686:errorcluster, 3:w687:refnum<k16>)  [unwired: 1 in]
            }
          }
          n188 = Select(t=FALSE, s=w662, f=TRUE) -> (s? t:f=w659:bool)
          "UDP_Out Status" <- w659
          n189 = node-c288() -> ()  [unwired: 1 in, 1 out]
          n190 = Unbundle(w656) -> ("status"=w657:bool)  [unwired: 2 out]
          n191 = Compound Arithmetic op=OR(w657, w654) -> (w655:bool)
        }
        n192 = node-c288(w651) -> ()  [unwired: 1 out]
        n193 = UDP Close(connection ID=w644, 8:w643) -> (error out=→"UDP_Out_Error Out":errorcluster)  [unwired: 1 out]
        n194 = Wait (ms)(milliseconds to wait=u32 1000) -> ()  [unwired: 1 out]
      }
      n195 = while {
        tunnel: w56 -> [w115]
        tunnel: w55 -> [w114]
        stop <- w118 stop-if-true
        # "Must delay to avoid 100% CPU on cRIO"
        # "TCP Loop writing to FISH Tank"
        n196 = TCP Open Connection(address="192.168.101.110", remote port or service name=u16 3502) -> (connection ID=w121:refnum<k5>, error out=w116:errorcluster)  [unwired: 3 in]
        n197 = case shown="No Error" w116 {
          selector: w116 -> [w126 w153]
          tunnel: w121 -> [w131 w154]
          tunnel: [w130 w154] -> w120
          tunnel: [w129 w153] -> w119
          tunnel: [w128 FALSE] -> w118
          tunnel: w115 -> [w125 _]
          tunnel: w114 -> [w124 _]
          frame No Error {
            n198 = node-c288() -> (w133:T1)  [unwired: 4 in]
            n199 = timed-loop {
              tunnel: w131 -> [w147]
              tunnel: w126 -> [w146]
              tunnel: [w145] -> w130
              tunnel: [w144] -> w129
              tunnel: [w134] -> w128
              shift-right: [w138] -> _
              shift-left: FALSE -> [w141]
              timing: w133 -> [_]
              timing-out: [_] -> w132
              tunnel: w125 -> [w137]
              tunnel: w124 -> [w136]
              stop <- w142 stop-if-true
              w134 = FALSE
              n200 = node-c288() -> ()  [unwired: 1 in, 1 out]
              n201 = Dequeue Element(queue=w137, error in (no error)=w136) -> (element=w135:string)  [unwired: 1 in, 3 out]
              n202 = Select(t=FALSE, s=w141, f=TRUE) -> (s? t:f=w138:bool)
              "TCP packet\nSend To FISH" <- w138
              n203 = TCP Write(connection ID=w147, data in=w135, error in (no error)=w146) -> (connection ID out=w145:refnum<k5>, error out=w144:errorcluster)  [unwired: 1 in, 1 out]
              n204 = Unbundle(w144) -> ("status"=w143:bool)  [unwired: 2 out]
              n205 = node-c288() -> ()  [unwired: 1 in, 1 out]
              n206 = Compound Arithmetic op=OR(w143, w134) -> (w142:bool)
            }
            n207 = node-c288(w132) -> ()  [unwired: 1 out]
          }
          frame Error {
          }
        }
        n208 = TCP Close Connection(connection ID=w120, error in (no error)=w119) -> (error out=→"FISH TCP Error Out":errorcluster)  [unwired: 1 in, 1 out]
        n209 = Wait (ms)(milliseconds to wait=u32 1000) -> ()  [unwired: 1 out]
      }
      n210 = while {
        tunnel: w54 -> [w73]
        tunnel: w53 -> [w72]
        stop <- w76 stop-if-true
        # "Must delay to avoid 100% CPU on cRIO"
        # "TCP Loop writing to SEPTIC Tank"
        n211 = TCP Open Connection(address="192.168.101.108", remote port or service name=u16 3502) -> (connection ID=w79:refnum<k5>, error out=w74:errorcluster)  [unwired: 3 in]
        n212 = case shown="No Error" w74 {
          selector: w74 -> [w84 w111]
          tunnel: w79 -> [w89 w112]
          tunnel: [w88 w112] -> w78
          tunnel: [w87 w111] -> w77
          tunnel: [w86 FALSE] -> w76
          tunnel: w73 -> [w83 _]
          tunnel: w72 -> [w82 _]
          frame No Error {
            n213 = node-c288() -> (w91:T1)  [unwired: 4 in]
            n214 = timed-loop {
              tunnel: w89 -> [w105]
              tunnel: w84 -> [w104]
              tunnel: [w103] -> w88
              tunnel: [w102] -> w87
              tunnel: [w92] -> w86
              shift-right: [w96] -> _
              shift-left: FALSE -> [w99]
              timing: w91 -> [_]
              timing-out: [_] -> w90
              tunnel: w83 -> [w95]
              tunnel: w82 -> [w94]
              stop <- w100 stop-if-true
              w92 = FALSE
              n215 = node-c288() -> ()  [unwired: 1 in, 1 out]
              n216 = Dequeue Element(queue=w95, error in (no error)=w94) -> (element=w93:string)  [unwired: 1 in, 3 out]
              n217 = Select(t=FALSE, s=w99, f=TRUE) -> (s? t:f=w96:bool)
              "TCP packet\nSend To SEPTIC" <- w96
              n218 = TCP Write(connection ID=w105, data in=w93, error in (no error)=w104) -> (connection ID out=w103:refnum<k5>, error out=w102:errorcluster)  [unwired: 1 in, 1 out]
              n219 = Unbundle(w102) -> ("status"=w101:bool)  [unwired: 2 out]
              n220 = node-c288() -> ()  [unwired: 1 in, 1 out]
              n221 = Compound Arithmetic op=OR(w101, w92) -> (w100:bool)
            }
            n222 = node-c288(w90) -> ()  [unwired: 1 out]
          }
          frame Error {
          }
        }
        n223 = TCP Close Connection(connection ID=w78, error in (no error)=w77) -> (error out=→"SEPTIC TCP Error Out":errorcluster)  [unwired: 1 in, 1 out]
        n224 = Wait (ms)(milliseconds to wait=u32 1000) -> ()  [unwired: 1 out]
      }
      n225 = while {
        stop <- FALSE stop-if-true
        n226 = node-c288() -> (w375:T1)  [unwired: 4 in]
        n227 = Create Network Stream Reader Endpoint(7:10 ("reader buffer size"), 9:T4 {"Message"="", "Message Data"=variant} ("Message Cluster"), 11:"/command/reader/CO" ("reader url")) -> (0:w381:errorcluster, 3:w382:refnum<k21>)  [unwired: 4 in]
        n228 = timed-loop "Host->Target Command Reader" {
          shift-right: [w392] -> w379
          shift-left: w381 -> [w395]
          shift-right: [w393] -> w378
          shift-left: w382 -> [w394]
          tunnel: [TRUE] -> _
          timing: w375 -> [_]
          timing-out: [_] -> w374
          stop <- w386 stop-if-true
          # "Receive Commands from Host VI"
          n229 = node-c288() -> ()  [unwired: 1 in, 1 out]
          n230 = shared-variable-read(w394, w395) -> (w393:refnum<k21>, w388:errorcluster, w390:bool, w391:T4)  [unwired: 1 in]
          n231 = Or(x=w390, y=w388) -> (x .or. y?=w389:bool)
          n232 = case shown="False" w389 {
            selector: w389 -> [_ w427]
            tunnel: w388 -> [w403 w428]
            tunnel: [w402 w428] -> w392
            tunnel: w391 -> [w401 _]
            tunnel: [w398 w427] -> w386
            frame False {
              n233 = Unbundle By Name(w401) -> ("Message"=w400:string, "Message Data"=w399:variant)
              n234 = case shown="\"CO CAL\"" w400 {
                tunnel: w403 -> [w407 w412 w414 w420 w426]
                tunnel: [w404 w409 w414 w419 w425] -> w402
                tunnel: w399 -> [w408 w413 _ w418 w424]
                tunnel: [_ _ TRUE _ _] -> w398
                frame "Stop File Write" {
                  n235 = Variant To Data(error in=w407, type=FALSE, Variant=w408) -> (data=→"Stop File Write":bool, error out=w404:errorcluster)
                }
                frame "Flight Number" {
                  n236 = Variant To Data(error in=w412, type="", Variant=w413) -> (data=→"Flight Number":string, error out=w409:errorcluster)
                }
                frame "Stop", Default {
                }
                frame "CO CAL" {
                  n237 = Variant To Data(error in=w420, type=FALSE, Variant=w418) -> (data=→"CO CAL":bool, error out=w419:errorcluster)
                }
                frame "CO Vacuum" {
                  n238 = Variant To Data(error in=w426, type=FALSE, Variant=w424) -> (data=w421:bool, error out=w425:errorcluster)
                  "CO Vacuum" <- w421
                  n239 = Boolean To (0,1)(Boolean=w421) -> (0, 1=→"CO Vacuum?":i16)
                  n240 = shared-variable "NI-cRIO9022-019C2C95\\Mod6\\DO5"(w421) -> ()  [unwired: 1 in, 1 out]
                }
              }
            }
            frame True {
            }
          }
          n241 = node-c288() -> ()  [unwired: 1 in, 1 out]
        }
        n242 = node-c288(w374) -> ()  [unwired: 1 out]
        n243 = Destroy Stream Endpoint(8:w379, 11:w378) -> (0:→"error out":errorcluster)
        n244 = Wait (ms)(milliseconds to wait=u32 1000) -> ()  [unwired: 1 out]
      }
      n245 = node-c288(w42) -> ()  [unwired: 1 out]
    }
    frame Error {
    }
  }
  n246 = disable-structure shown="Enabled" {
    frame Disabled {
      n247 = while {
        stop <- FALSE stop-if-true
        # "Must delay to avoid 100% CPU on cRIO"
        # "CO Control Data Loop"
        n248 = call <vilib>:"TCP Listen.vi"("port"=u16 1002) -> ("error out"=w702:errorcluster, "connection ID"=w703:refnum<k5>)  [unwired: 6 in, 3 out]
        n249 = node-c288() -> (w706:T1)  [unwired: 4 in]
        n250 = timed-loop {
          timing: w706 -> [_]
          timing-out: [_] -> w705
          tunnel: w703 -> [w723]
          tunnel: w702 -> [w722]
          tunnel: [w712] -> w701
          tunnel: [w711] -> w700
          stop <- w711 stop-if-true
          n251 = node-c288() -> ()  [unwired: 1 in, 1 out]
          n252 = TCP Read(connection ID=w723, bytes to read=4, error in (no error)=w722) -> (connection ID out=w720:refnum<k5>, data out=w717:string, error out=w719:errorcluster)  [unwired: 2 in]
          n253 = Type Cast(type=0, x=w717) -> (*(type *) &x=w716:i32)
          n254 = TCP Read(connection ID=w720, bytes to read=w716, error in (no error)=w719) -> (connection ID out=w712:refnum<k5>, data out=w713:string, error out=w711:errorcluster)  [unwired: 2 in]
          "Control data out" <- w713
          n255 = Spreadsheet String To Array(delimiter (Tab)=",", format string="%b", spreadsheet string=w713, array type (2D Dbl)=i32[] []) -> (array=w710:i32[])
          "Control data" <- w710
          n256 = Index Array(array=w710) -> (element #2=w708:i32)  [unwired: 2 in, 1 out]
          n257 = Not Equal To 0?(x=w708) -> (x != 0?=w707:bool)
          n258 = shared-variable "NI-cRIO9022-019C2C95\\Mod6\\DO5"(w707) -> ()  [unwired: 1 in, 1 out]
          n259 = node-c288() -> ()  [unwired: 1 in, 1 out]
        }
        n260 = Wait (ms)(milliseconds to wait=u32 1000) -> ()  [unwired: 1 out]
        n261 = node-c288(w705) -> ()  [unwired: 1 out]
        n262 = TCP Close Connection(connection ID=w701, error in (no error)=w700) -> ()  [unwired: 1 in, 2 out]
      }
    }
    frame Enabled {
    }
  }
  n263 = VISA Close(VISA resource name=w14, error in (no error)=w15) -> (error out=→"Serial VISA error":errorcluster)
